vi "BRig_dataTrial_sCue.vi"() -> (2 "output_sCue":i32)   [LabVIEW 2014]
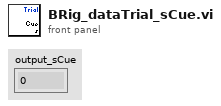
[diagram p1: front panel]
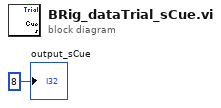
[diagram p0: block diagram]
diagram:
  "output_sCue" <- 8 ("output_iBlock")
